vi "Front Panel.vi"(11 "GUI In":refnum<class "PAS Control.lvclass">) -> ()   [LabVIEW 2015, in "PAS Control.lvclass"]
uses:
  PAS Control.lvclass
  Interface/Controls/PAS_MFC_SP.ctl
  Interface/Controls/pasCellTEC.ctl
  Interface/Controls/pasTECen.ctl
  Interface/Controls/pasLasCtl.ctl
  Utilities/FPGA/Controls/FPGAConfig.ctl
  Reusable/PAS/Main/Controls/Laser Modulation.ctl
  Reusable/GUI/GUI.lvclass/GUI.ctl
  Reusable/Observer/Observer.lvclass/Observer.ctl
  Data/cPAS Data.lvclass
  Data/cPAS Data.lvclass/cPAS Data.ctl
  Data/cPAS Cell Data/cPAS Cell Data.lvclass
  Data/Read Serial Data.vi
  Reusable/GUI/Accessors/Read RegEvent.vi
  Reusable/Observer/Read Data Queue.vi
  Reusable/PAS/Data/Main/Read CellData.vi
  Data/Read Thum.vi
  Reusable/PAS/Data/Cell/Read houseKeeping.vi
  Data/Read T2_cell.vi
  Reusable/Data/Data.lvclass
  Reusable/PAS/Data/Cell/PAS Cell Data.lvclass
panel:
  in  "Speaker DC":cluster{"Length":dbl, "Period":dbl}
  out "tecT":cluster{"pasTte 2":sgl, "pasTte":sgl} caption="TEC Temperature\n(degC)" {"pasTte" format="%#.2f"; "pasTte 2" format="%#.2f"}
  in  "pasLasCtl":T1 caption="Laser Control" {"Laser Output"."Span"."ch 5" min=0 max=20; "Laser Output"."Span"."ch 4" min=0 max=20; "Laser Output"."Span"."ch 3" min=0 max=20; "Laser Output"."Span"."ch 2" min=0 max=20; "Laser Output"."Span"."ch 1" min=0 max=20; "f0"."Cell 1" max=2000 step=1; "f0"."Cell 2" max=2000 step=1; "f0"."Cell 3" max=2000 step=1; "f0"."Cell 4" max=2000 step=1; "f0"."Cell 5" max=2000 step=1}
  out "PASCellT2":T4 caption="Thermistor Cell Temperature (degC)" {"Cell 5" format="%.2f"; "Cell 4" format="%.2f"; "Cell 3" format="%.2f"; "Cell 2" format="%.2f"; "Cell 1" format="%.2f"}
  out "tecP":sgl caption="TEC Power (%)" format="%#.2f"
  in  "pas::rhctl":bool caption="RH Control"
  in  "pas::rh":dbl caption="RH (%)"
  in  "ptecHumEn":bool caption="Enable"
  in  "pas::satT":sgl caption="T(degC)"
  out "PASCellT":T5 caption="TEC Thermistor Cell Temperature (degC)" {"Cell 5" format="%.2f"; "Cell 4" format="%.2f"; "Cell 3" format="%.2f"; "Cell 2" format="%.2f"; "Cell 1" format="%.2f"}
  out "pasRH":T6 caption="Vaisala Data" {"c 5"."TRH" format="%#.2f"; "c 5"."RH" format="%#.2f"; "c 4"."TRH" format="%#.2f"; "c 4"."RH" format="%#.2f"; "c 3"."TRH" format="%#.2f"; "c 3"."RH" format="%#.2f"; "c 2"."TRH" format="%#.2f"; "c 2"."RH" format="%#.2f"; "c 1"."TRH" format="%#.2f"; "c 1"."RH" format="%#.2f"}
  out "pasACat":T7 caption="Alicat Data" {"c 5 2"."P" format="%.2f"; "c 5 2"."T" format="%.2f"; "c 5 2"."Q" format="%.2f"; "c 4"."P" format="%.2f"; "c 4"."T" format="%.2f"; "c 4"."Q" format="%.2f"; "c 3"."P" format="%.2f"; "c 3"."T" format="%.2f"; "c 3"."Q" format="%.2f"; "c 2"."P" format="%.2f"; "c 2"."T" format="%.2f"; "c 2"."Q" format="%.2f"; "c 1"."P" format="%.2f"; "c 1"."T" format="%.2f"; "c 1"."Q" format="%.2f"}
  in  "pasTECEn":T8 caption="Enable TECs"
  in  "pasTcell":T9 caption="Temperature \n (degC)"
  in  "pasFlows":T10 caption="Flow Rate Setpoint (LPM)" {"Cell 5" min=0 max=5; "Cell 4" min=0 max=5; "Cell 3" min=0 max=5; "Cell 2" min=0 max=5; "Cell 1" min=0 max=5}
  in  "pasTteSP":sgl caption="TEC Setpoint \n(degC)" format="%#.2f"
  out "Thum":sgl caption="Tsat\n(degC)" format="%#.2g"
  # "PAS Housekeeping Data"
  # "PAS Controls"
  # "TEC Temperature Control"
  # "RH Control"
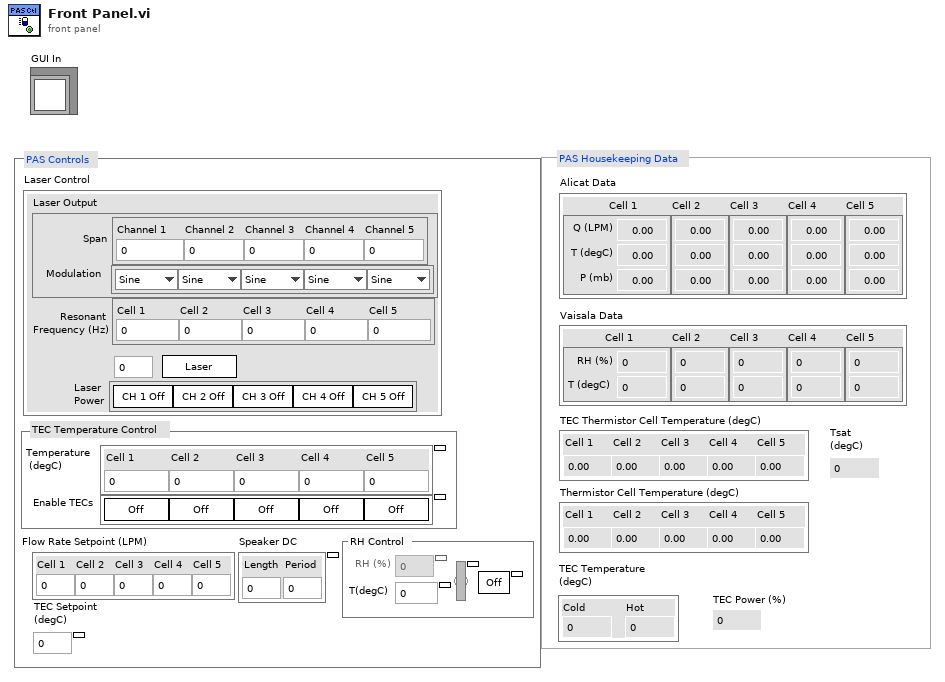
[diagram p1: front panel]
types:
  T1 = typedef "pasLasCtl.ctl" = cluster{"Laser Output":T2, "f0":cluster{"Cell 1":u16, "Cell 2":u16, "Cell 3":u16, "Cell 4":u16, "Cell 5":u16}, "drive":bool, "Speake Voltage":sgl, "lasPower":cluster{"ch 1":bool, "ch 2":bool, "ch 3":bool, "ch 4":bool, "ch 5":bool}}
  T2 = typedef "FPGAConfig.ctl" = cluster{"Span":cluster{"ch 1":sgl, "ch 2":sgl, "ch 3":sgl, "ch 4":sgl, "ch 5":sgl}, "mod":cluster{"ch 1":T3, "ch 2":T3, "ch 3":T3, "ch 4":T3, "ch 5":T3}}
  T3 = typedef "Laser Modulation.ctl" = enum8{"Sine", "Square"}
  T4 = cluster{"[0]":sgl, "[1]":sgl, "[2]":sgl, "[3]":sgl, "[4]":sgl}
  T5 = cluster{"ScaledData[0]":sgl, "ScaledData[1]":sgl, "ScaledData[2]":sgl, "ScaledData[3]":sgl, "ScaledData[4]":sgl}
  T6 = cluster{"c 1":cluster{"RH":sgl, "TRH":sgl}, "c 2":cluster{"RH":sgl, "TRH":sgl}, "c 3":cluster{"RH":sgl, "TRH":sgl}, "c 4":cluster{"RH":sgl, "TRH":sgl}, "c 5":cluster{"RH":sgl, "TRH":sgl}}
  T7 = cluster{"c 1":cluster{"Q":sgl, "T":sgl, "P":sgl}, "c 2":cluster{"Q":sgl, "T":sgl, "P":sgl}, "c 3":cluster{"Q":sgl, "T":sgl, "P":sgl}, "c 4":cluster{"Q":sgl, "T":sgl, "P":sgl}, "c 5 2":cluster{"Q":sgl, "T":sgl, "P":sgl}}
  T8 = typedef "pasTECen.ctl" = cluster{"Cell 1":bool, "Cell 2":bool, "Cell 3":bool, "Cell 4":bool, "Cell 5":bool}
  T9 = typedef "pasCellTEC.ctl" = cluster{"Cell 1":sgl, "Cell 2":sgl, "Cell 3":sgl, "Cell 4":sgl, "Cell 5":sgl}
  T10 = typedef "PAS_MFC_SP.ctl" = cluster{"Cell 1":sgl, "Cell 2":sgl, "Cell 3":sgl, "Cell 4":sgl, "Cell 5":sgl}
  T11 = cluster{"ch 1":bool, "ch 2":bool, "ch 3":bool, "ch 4":bool, "ch 5":bool}
  T12 = cluster{"Array of Boolean[0]":bool, "Array of Boolean[1]":bool, "Array of Boolean[2]":bool, "Array of Boolean[3]":bool, "Array of Boolean[4]":bool}
  T13 = cluster{"T":sgl, "TRH":sgl, "RH":sgl, "laserRMS":sgl}
  T14 = cluster{"Array of Single[0]":sgl, "Array of Single[1]":sgl, "Array of Single[2]":sgl, "Array of Single[3]":sgl, "Array of Single[4]":sgl}
  T15 = cluster{"[0]":cluster{"Q":sgl, "T":sgl, "P":sgl}, "[1]":cluster{"Q":sgl, "T":sgl, "P":sgl}, "[2]":cluster{"Q":sgl, "T":sgl, "P":sgl}, "[3]":cluster{"Q":sgl, "T":sgl, "P":sgl}, "[4]":cluster{"Q":sgl, "T":sgl, "P":sgl}}
  T16 = cluster{"Input 1":sgl, "Input 2":sgl, "Power":sgl}
  T17 = cluster{"Array of UInt8[0]":u8, "Array of UInt8[1]":u8, "Array of UInt8[2]":u8, "Array of UInt8[3]":u8, "Array of UInt8[4]":u8}
  T18 = cluster{"[0]":cluster{"RH":sgl, "TRH":sgl}, "[1]":cluster{"RH":sgl, "TRH":sgl}, "[2]":cluster{"RH":sgl, "TRH":sgl}, "[3]":cluster{"RH":sgl, "TRH":sgl}, "[4]":cluster{"RH":sgl, "TRH":sgl}}
  T19 = cluster{"Array of UInt16[0]":u16, "Array of UInt16[1]":u16, "Array of UInt16[2]":u16, "Array of UInt16[3]":u16, "Array of UInt16[4]":u16}
  T20 = cluster{"ch 1":sgl, "ch 2":sgl, "ch 3":sgl, "ch 4":sgl, "ch 5":sgl}
  T21 = cluster{"ch 1":T3, "ch 2":T3, "ch 3":T3, "ch 4":T3, "ch 5":T3}
  T22 = cluster{"Cell 1":u16, "Cell 2":u16, "Cell 3":u16, "Cell 4":u16, "Cell 5":u16}
  T23 = enum8{"Enabled", "Disabled", "Disabled and Grayed Out"}
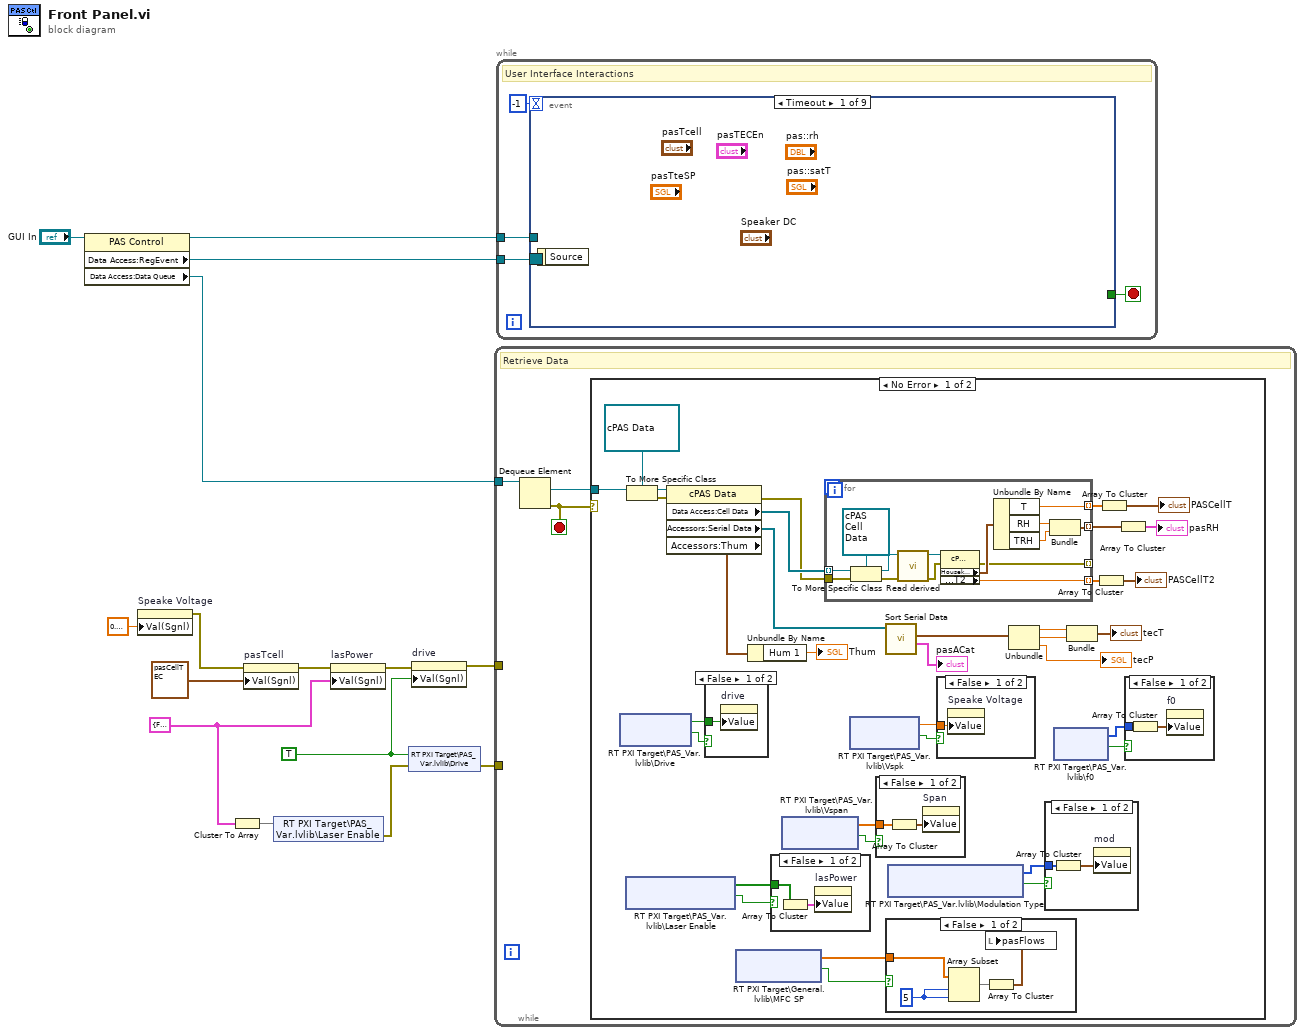
[diagram p0: block diagram]
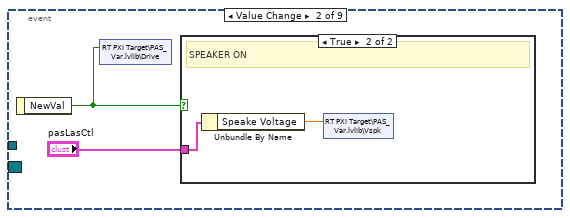
[diagram p10: hidden frame]
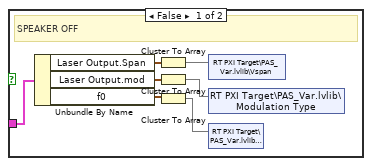
[diagram p11: hidden frame]
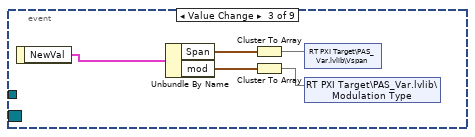
[diagram p12: hidden frame]
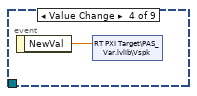
[diagram p13: hidden frame]
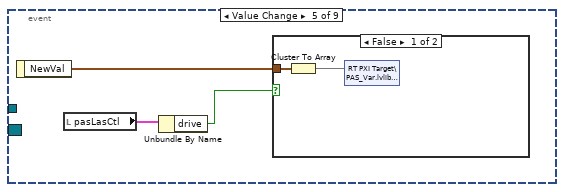
[diagram p14: hidden frame]
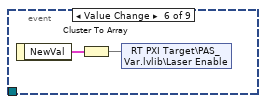
[diagram p16: hidden frame]
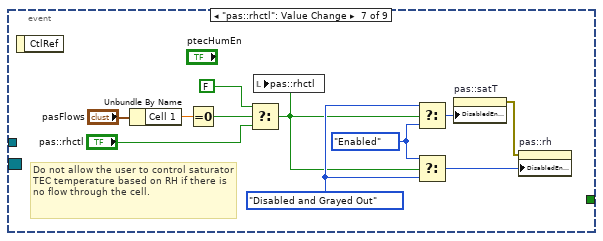
[diagram p17: hidden frame]
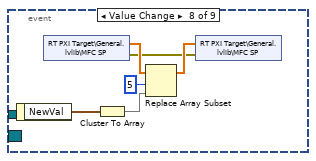
[diagram p18: hidden frame]
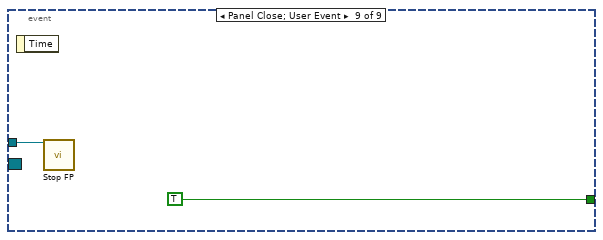
[diagram p19: hidden frame]
diagram:
  w5 = TRUE ("Value (Signaling)")
  w3 = T11 {"ch 1"=FALSE, "ch 2"=FALSE, "ch 3"=FALSE, "ch 4"=FALSE, "ch 5"=FALSE} ("Value (Signaling)")
  n1 = property class="PAS Control"(reference="GUI In") -> (reference out=w12:refnum<class "PAS Control.lvclass">, "Data Access:RegEvent"=w15:refnum<event-registration>, "Data Access:Data Queue"=w14:refnum<queue>)  [unwired: 1 in, 1 out]
  n2 = property on="Speake Voltage" class="DigNum (strict)"("Val(Sgnl)"=sgl 0.9 ("Value (Signaling)")) -> (error out=w9:errorcluster)  [unwired: 2 in, 1 out]
  n3 = Cluster To Array(cluster=w3) -> (array=w2:bool[])
  n4 = property on="pasTcell" class="Clust (strict)"(error in=w9, "Val(Sgnl)"=T9 {"Cell 1"=19.0, "Cell 2"=19.0, "Cell 3"=19.0, "Cell 4"=19.0, "Cell 5"=20.0} ("Value (Signaling)")) -> (error out=w8:errorcluster)  [unwired: 1 in, 1 out]
  n5 = shared-variable "RT PXI Target\\PAS_Var.lvlib\\Laser Enable"(w2) -> (error out=w1:errorcluster)  [unwired: 1 in]
  n6 = property on="lasPower" class="Clust (strict)"(error in=w8, "Val(Sgnl)"=w3) -> (error out=w7:errorcluster)  [unwired: 1 in, 1 out]
  n7 = shared-variable "RT PXI Target\\PAS_Var.lvlib\\Drive"(w5, error in=w1) -> (error out=w4:errorcluster)
  n8 = property on="drive" class="Bool (strict)"(error in=w7, "Val(Sgnl)"=w5) -> (error out=w6:errorcluster)  [unwired: 1 in, 1 out]
  n9 = while {
    tunnel: w14 -> [w18]
    tunnel: w6 -> [_]
    tunnel: w4 -> [_]
    stop <- w17 stop-if-true
    # "Retrieve Data"
    n10 = Dequeue Element(queue=w18) -> (element=w16:refnum<data-value>, error out=w17:errorcluster)  [unwired: 2 in, 2 out]
    n11 = case shown="No Error" w17 {
      tunnel: w16 -> [w41 _]
      frame No Error {
        n12 = shared-variable "RT PXI Target\\PAS_Var.lvlib\\Drive"() -> (w27:bool, w28:bool)  [unwired: 2 in, 1 out]
        n13 = shared-variable "RT PXI Target\\PAS_Var.lvlib\\Laser Enable"() -> (w21:bool[], w22:bool)  [unwired: 2 in, 1 out]
        n14 = To More Specific Class(target class=refnum<data-value> refnum ("DVR"), reference=w41) -> (specific class reference=w39:refnum<data-value>, error out=w38:errorcluster)  [unwired: 1 in]
        n15 = property class="cPAS Data"(reference=w39, error in=w38) -> (error out=w46:errorcluster, "Data Access:Cell Data"=w47:refnum<class "PAS Cell Data.lvclass">[], "Accessors:Serial Data"=w45:refnum<class "Data.lvclass">[], "Accessors:Thum"=w43:cluster{"Hum 1":sgl, "Hum 2":sgl})  [unwired: 1 out]
        n16 = case shown="False" w28 {
          tunnel: w27 -> [w63 _]
          frame False {
            n17 = property on="drive" class="Bool (strict)"("Value"=w63) -> ()  [unwired: 2 in, 2 out]
          }
          frame True {
          }
        }
        n18 = shared-variable "RT PXI Target\\General.lvlib\\MFC SP"() -> (w20:sgl[], w19:bool)  [unwired: 2 in, 1 out]
        n19 = Unbundle By Name(w43) -> ("Hum 1"=→"Thum":sgl)
        n20 = case shown="False" w22 {
          tunnel: w21 -> [w59 _]
          frame False {
            n21 = Array To Cluster(array=w59) -> (cluster=w58:T12)
            n22 = property on="lasPower" class="Clust (strict)"("Value"=w58) -> ()  [unwired: 2 in, 2 out]
          }
          frame True {
          }
        }
        n23 = shared-variable "RT PXI Target\\PAS_Var.lvlib\\Vspan"() -> (w24:sgl[], w23:bool)  [unwired: 2 in, 1 out]
        n24 = for {
          tunnel: w47 -> [w71] mode=indexing
          tunnel: [w78] -> w50 mode=indexing
          tunnel: [w79] -> w51 mode=indexing
          tunnel: w46 -> [w74]
          tunnel: [w69] -> _ mode=indexing
          tunnel: [w68] -> w49 mode=indexing
          n25 = To More Specific Class(target class=refnum<class "cPAS Cell Data.lvclass"> refnum ("cPAS Cell"), reference=w71, error in=w74) -> (specific class reference=w70:refnum<class "cPAS Cell Data.lvclass">, error out=w73:errorcluster)
          n26 = call "Read derived.vi"("error in"=w73, "PAS Cell Data in"=w70) -> ("error out"=w81:errorcluster, "PAS Cell Data out"=w76:refnum<class "cPAS Cell Data.lvclass">)  [unwired: 7 in, 1 out]
          n27 = property class="cPAS Cell"(reference=w76, error in=w81) -> (error out=w69:errorcluster, "Housekeeping"=w75:T13, "Data Access:T2"=w68:sgl)  [unwired: 1 out]
          n28 = Unbundle By Name(w75) -> ("T"=w78:sgl, "RH"=w77:sgl, "TRH"=w80:sgl)
          n29 = Bundle("RH"=w77, "TRH"=w80) -> (w79:cluster{"RH":sgl, "TRH":sgl})  [unwired: 1 in]
        }
        n30 = shared-variable "RT PXI Target\\PAS_Var.lvlib\\Vspk"() -> (w26:sgl, w25:bool)  [unwired: 2 in, 1 out]
        n31 = case shown="False" w23 {
          tunnel: w24 -> [w60 _]
          frame False {
            n32 = Array To Cluster(array=w60) -> (cluster=w61:T14)
            n33 = property on="Span" class="Clust (strict)"("Value"=w61) -> ()  [unwired: 2 in, 2 out]
          }
          frame True {
          }
        }
        n34 = call "Sort Serial Data.vi"("SerialData"=w45) -> ("acatDataOut"=→"pasACat":T15, "TEC Data"=w37:T16)  [unwired: 8 in, 1 out]
        n35 = case shown="False" w19 {
          tunnel: w20 -> [w55 _]
          frame False {
            w54 = 5 ("length")
            n36 = Array Subset(array=w55, index=w54, length=w54) -> (w56:sgl[])
            n37 = Array To Cluster(array=w56) -> (cluster=w57:T4)
            n38 = local write "pasFlows"(w57) -> ()
          }
          frame True {
          }
        }
        n39 = shared-variable "RT PXI Target\\PAS_Var.lvlib\\Modulation Type"() -> (w29:u8[], w32:bool)  [unwired: 2 in, 1 out]
        n40 = case shown="False" w25 {
          tunnel: w26 -> [w62 _]
          frame False {
            n41 = property on="Speake Voltage" class="DigNum (strict)"("Value"=w62) -> ()  [unwired: 2 in, 2 out]
          }
          frame True {
          }
        }
        n42 = Unbundle(w37) -> ("Input 1"=w35:sgl, "Input 2"=w34:sgl, "Power"=→"tecP":sgl)
        n43 = case shown="False" w32 {
          tunnel: w29 -> [w67 _]
          frame False {
            n44 = Array To Cluster(array=w67) -> (cluster=w66:T17)
            n45 = property on="mod" class="Clust (strict)"("Value"=w66) -> ()  [unwired: 2 in, 2 out]
          }
          frame True {
          }
        }
        n46 = shared-variable "RT PXI Target\\PAS_Var.lvlib\\f0"() -> (w30:u16[], w31:bool)  [unwired: 2 in, 1 out]
        n47 = Bundle("Input 1"=w35, "Input 2"=w34) -> (→"tecT":cluster{"Input 1":sgl, "Input 2":sgl})  [unwired: 1 in]
        n48 = Array To Cluster(array=w49) -> (cluster=→"PASCellT2":T4)
        n49 = Array To Cluster(array=w50) -> (cluster=→"PASCellT":T4)
        n50 = Array To Cluster(array=w51) -> (cluster=→"pasRH":T18)
        n51 = case shown="False" w31 {
          tunnel: w30 -> [w65 _]
          frame False {
            n52 = Array To Cluster(array=w65) -> (cluster=w64:T19)
            n53 = property on="f0" class="Clust (strict)"("Value"=w64) -> ()  [unwired: 2 in, 2 out]
          }
          frame True {
          }
        }
      }
      frame Error {
      }
    }
  }
  n54 = while {
    tunnel: w15 -> [w83]
    tunnel: w12 -> [w82]
    stop <- w85 stop-if-true
    # "User Interface Interactions"
    n55 = event shown="[0] Timeout" {
      selector: w83 -> [_ _ _ _ _ _ _ _ _]
      dyn-events: _ -> [_ _ _ _ _ _ _ _ _]
      timeout: -1 -> [_ _ _ _ _ _ _ _ _]
      tunnel: [_ _ _ _ _ _ _ _ TRUE] -> w85
      tunnel: w82 -> [_ _ _ _ _ _ _ _ w127]
      event Timeout {
        n56 = event-data() -> ()  [unwired: 1 in, 1 out]
      }
      event Value Change {
        n57 = event-data() -> ("NewVal"=w87:bool)  [unwired: 1 in]
        n58 = shared-variable "RT PXI Target\\PAS_Var.lvlib\\Drive"(w87) -> ()  [unwired: 1 in, 1 out]
        n59 = case shown="True" w87 {
          tunnel: "pasLasCtl" -> [w94 w96]
          frame False {
            # "SPEAKER OFF"
            n60 = Unbundle By Name(w94) -> ("Laser Output.Span"=w89:T20, "Laser Output.mod"=w90:T21, "f0"=w92:T22)
            n61 = Cluster To Array(cluster=w89) -> (array=w88:sgl[])
            n62 = Cluster To Array(cluster=w90) -> (array=w91:T3[])
            n63 = Cluster To Array(cluster=w92) -> (array=w93:u16[])
            n64 = shared-variable "RT PXI Target\\PAS_Var.lvlib\\Vspan"(w88) -> ()  [unwired: 1 in, 1 out]
            n65 = shared-variable "RT PXI Target\\PAS_Var.lvlib\\Modulation Type"(w91) -> ()  [unwired: 1 in, 1 out]
            n66 = shared-variable "RT PXI Target\\PAS_Var.lvlib\\f0"(w93) -> ()  [unwired: 1 in, 1 out]
          }
          frame True {
            # "SPEAKER ON"
            n67 = Unbundle By Name(w96) -> ("Speake Voltage"=w95:sgl)
            n68 = shared-variable "RT PXI Target\\PAS_Var.lvlib\\Vspk"(w95) -> ()  [unwired: 1 in, 1 out]
          }
        }
      }
      event Value Change {
        n69 = event-data() -> ("NewVal"=w97:T2)  [unwired: 1 in]
        n70 = Unbundle By Name(w97) -> ("Span"=w100:T20, "mod"=w99:T21)
        n71 = Cluster To Array(cluster=w100) -> (array=w101:sgl[])
        n72 = Cluster To Array(cluster=w99) -> (array=w98:T3[])
        n73 = shared-variable "RT PXI Target\\PAS_Var.lvlib\\Vspan"(w101) -> ()  [unwired: 1 in, 1 out]
        n74 = shared-variable "RT PXI Target\\PAS_Var.lvlib\\Modulation Type"(w98) -> ()  [unwired: 1 in, 1 out]
      }
      event Value Change {
        n75 = event-data() -> ("NewVal"=w102:sgl)  [unwired: 1 in]
        n76 = shared-variable "RT PXI Target\\PAS_Var.lvlib\\Vspk"(w102) -> ()  [unwired: 1 in, 1 out]
      }
      event Value Change {
        n77 = event-data() -> ("NewVal"=w105:T22)  [unwired: 1 in]
        n78 = local read "pasLasCtl"() -> (w104:T1)
        n79 = Unbundle By Name(w104) -> ("drive"=w103:bool)
        n80 = case shown="False" w103 {
          tunnel: w105 -> [w107 _]
          frame False {
            n81 = Cluster To Array(cluster=w107) -> (array=w106:u16[])
            n82 = shared-variable "RT PXI Target\\PAS_Var.lvlib\\f0"(w106) -> ()  [unwired: 1 in, 1 out]
          }
          frame True {
          }
        }
      }
      event Value Change {
        n83 = event-data() -> ("NewVal"=w108:T11)  [unwired: 1 in]
        n84 = Cluster To Array(cluster=w108) -> (array=w109:bool[])
        n85 = shared-variable "RT PXI Target\\PAS_Var.lvlib\\Laser Enable"(w109) -> ()  [unwired: 1 in, 1 out]
      }
      event "pas::rhctl": Value Change {
        w118 = T23."Disabled and Grayed Out" ("Disabled")
        w119 = T23."Enabled" ("Disabled")
        # "Do not allow the user to control saturator TEC temperature based on RH if there is no flow through the cell."
        n86 = event-data() -> ()  [unwired: 1 in, 1 out]
        n87 = Unbundle By Name("pasFlows") -> ("Cell 1"=w111:sgl)
        n88 = Equal To 0?(x=w111) -> (x = 0?=w115:bool)
        n89 = Select(t=FALSE, s=w115, f="pas::rhctl") -> (s? t:f=w113:bool)
        n90 = local write "pas::rhctl"(w113) -> ()
        n91 = Select(t=w118, s=w113, f=w119) -> (s? t:f=w117:T23)
        n92 = Select(t=w119, s=w113, f=w118) -> (s? t:f=w120:T23)
        n93 = property on="pas::satT" class="DigNum (strict)"("DisabledEnum"=w117) -> (error out=w116:errorcluster)  [unwired: 2 in, 1 out]
        n94 = property on="pas::rh" class="DigNum (strict)"(error in=w116, "DisabledEnum"=w120) -> ()  [unwired: 1 in, 2 out]
      }
      event Value Change {
        n95 = event-data() -> ("NewVal"=w125:T10)  [unwired: 1 in]
        n96 = shared-variable "RT PXI Target\\General.lvlib\\MFC SP"() -> (w126:sgl[], error out=w121:errorcluster)  [unwired: 1 in]
        n97 = Cluster To Array(cluster=w125) -> (array=w124:sgl[])
        n98 = Replace Array Subset(array=w126, new element=w124, index=5) -> (w122:sgl[])
        n99 = shared-variable "RT PXI Target\\General.lvlib\\MFC SP"(w122, error in=w121) -> ()  [unwired: 1 out]
      }
      event Panel Close; User Event {
        n100 = event-data() -> ()  [unwired: 1 in, 1 out]
        n101 = call-dynamic "Stop FP.vi"("GUI in"=w127) -> ()  [unwired: 9 in, 2 out]
      }
    }
  }
